vi "hdf5 convert folder of pngs.vi"() -> ()   [LabVIEW 2018]
panel:
  out "fopn png time":u32(graph)
  out "save time 2":u32(graph)
  out "error out":errorcluster
  in  "Chunk size":i32[](array[numeric])=[8, 8]
  in  "Compression Level (0-disabled)":i32=9
  in  "folder of images":path=path "C:/GEECS/data/Y2020/04-Apr/20_0420/scans/Scan022/SimCam"
  in  "File path":path=path "C:/GEECS/data/s22comp9ch8.hdf5"
  out "File Path":path=path "C:/GEECS/data/Y2020/04-Apr/20_0420/scans/Scan022/SimCam/Scan022_SimCam_100.png"
  # "17KB"
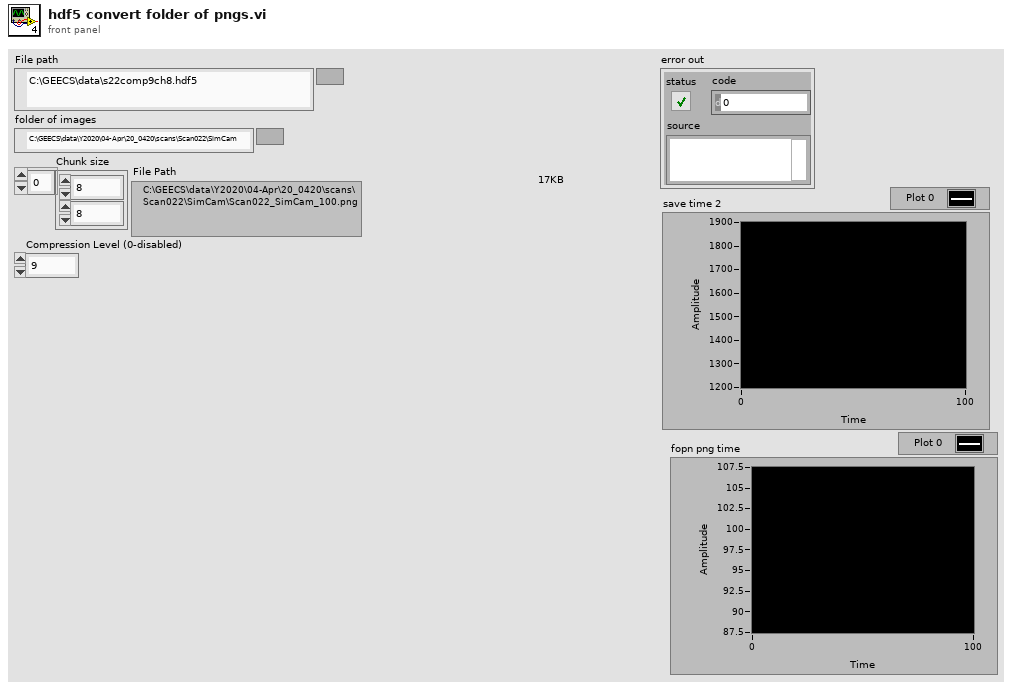
[diagram p1: front panel]
types:
  T1 = typedef "Image Type" = u32
  T2 = typedef "IMAQ Image.ctl" = refnum<image>
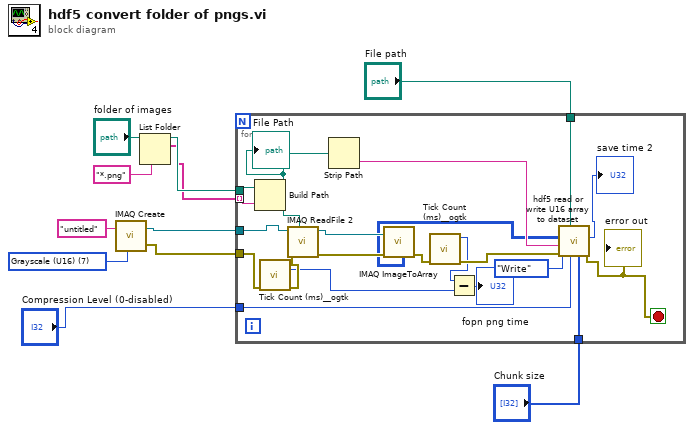
[diagram p0: block diagram]
diagram:
  w10 = T1 7 items=["Grayscale (U8)", "Grayscale (I16)", "Grayscale (SGL)", "Complex (CSG)", "RGB (U32)", "HSL (U32)", "RGB (U64)", "Grayscale (U16)"] ("Image Type")
  n1 = call "IMAQ Create"("Image Name"="untitled", "Image Type"=w10) -> ("New Image"=w9:T2, "error out"=w8:errorcluster)  [unwired: 3 in]
  n2 = List Folder(path="folder of images", pattern="*.png") -> (path out=w6:path, filenames=w5:string[])  [unwired: 2 in, 2 out]
  n3 = for {
    tunnel: w9 -> [w30]
    tunnel: w8 -> [w18]
    tunnel: "File path" -> [w27]
    tunnel: w6 -> [w26]
    tunnel: w5 -> [w25] mode=indexing
    tunnel: "Compression Level (0-disabled)" -> [w23]
    tunnel: "Chunk size" -> [w22]
    stop <- w21 stop-if-true
    n4 = Build Path(base path=w26, name or relative path=w25) -> (appended path=w24:path)
    "File Path" <- w24
    n5 = call <userlib>:"Tick Count (ms)__ogtk.vi"("error in (no error)"=w18) -> ("error out"=w17:errorcluster, "millisecond timer value"=w13:u32)  [unwired: 9 in]
    n6 = call "IMAQ ReadFile 2"("File Path"=w24, "error in (no error)"=w17, "Image"=w30) -> ("error out"=w32:errorcluster, "Image Out"=w31:T2)  [unwired: 4 in, 3 out]
    n7 = Strip Path(path=w24) -> (name=w28:string)  [unwired: 1 out]
    n8 = call "IMAQ ImageToArray"("error in (no error)"=w32, "Image"=w31) -> ("Image Pixels (U16)"=w20:u16[][], "error out"=w16:errorcluster)  [unwired: 2 in, 3 out]
    n9 = call <userlib>:"Tick Count (ms)__ogtk.vi"("error in (no error)"=w16) -> ("error out"=w15:errorcluster, "millisecond timer value"=w14:u32)  [unwired: 9 in]
    n10 = Subtract(x=w14, y=w13) -> (x-y=→"fopn png time":u32)
    n11 = call "hdf5 read or write U16 array to dataset.vi"("Chunk size"=w22, "Compression Level (0-disabled)"=w23, "File path"=w27, "error in"=w15, "Dataset name"=w28, "Data to write"=w20, "Operation"=enum32{"Write", "Read"}."Write") -> ("error out"=w21:errorcluster, "write time"=→"save time 2":u32)  [unwired: 2 in, 1 out]
    "error out" <- w21
  }
